vi "labview music visualizer.vi"() -> ()   [LabVIEW 2014]
uses:
  <vilib>/Analysis/3filter.llb/Filter Passband Type.ctl
  <vilib>/sound2/lvsound2.llb/Sampling Mode.ctl
  <vilib>/sound2/lvsound2.llb/Sound Output Write (DBL).vi
  <vilib>/Analysis/3filter.llb/Butterworth Filter (DBL).vi
  <vilib>/sound2/lvsound2.llb/Sound File Read (DBL).vi
  <vilib>/sound2/lvsound2.llb/Sound File Read Open.vi
  <vilib>/sound2/lvsound2.llb/Sound File Info (path).vi
  <vilib>/measure/maspectr.llb/FFT Power Spectrum and PSD for 1 Chan.vi
  <vilib>/measure/NI_MAPro.lvlib
  <vilib>/Analysis/NI_AALBase.lvlib
panel:
  out "Low Cutoff Freq, Hz":u32
  out "High Cutoff Freq, Hz":u32
  out "Filter Error!":bool
  in  "Filter Bands ,Hz":cluster{dbl, dbl}(slide)={22000.0, 10.0} scale=10.0..22000.0
  in  "Filter Type":T1=enum."Bandpass"
  out "Power Spectrum":waveform(dbl)(graph)
  out "digital spectrum":dbl[](array[slide]) scale=-42.0..6.0
  out "VU":dbl(knob) scale=-42.0..6.0
  out "Waveform":waveform(dbl)[](graph)
  in  "Stop":bool
  in  "Buffer Size (samples)":i32=2048
  in  "Music File":path=path "!!!"
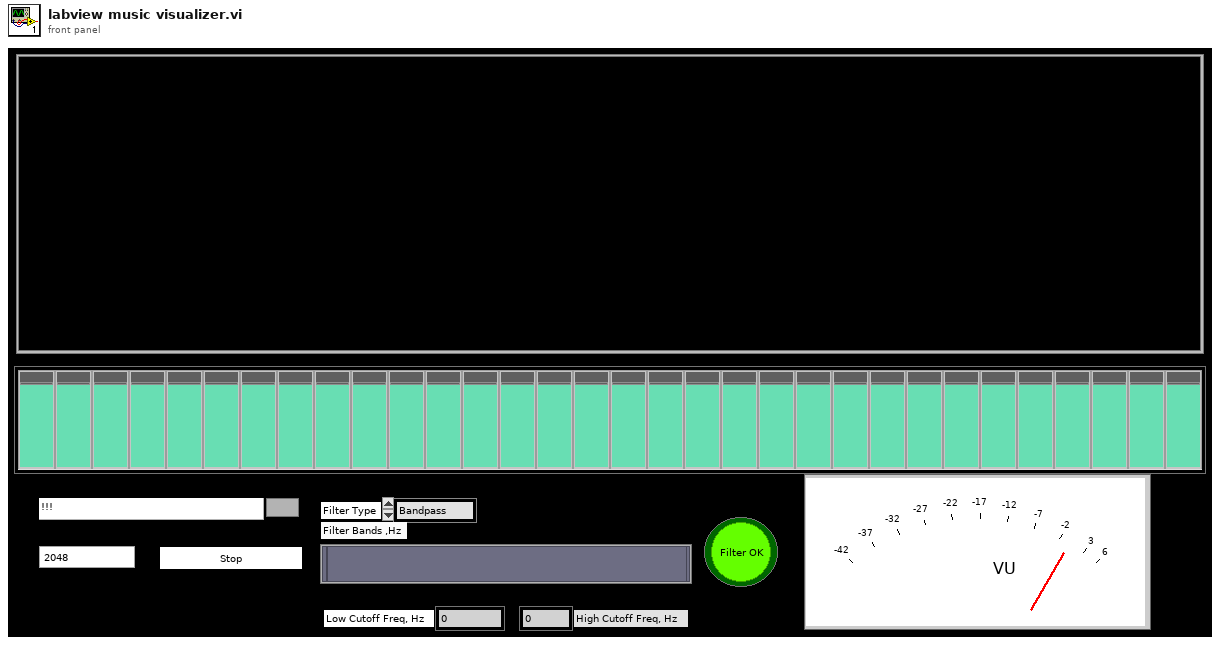
[diagram p1: front panel]
types:
  T1 = typedef "NI_AALBase.lvlib/Filter Passband Type.ctl" = enum32{"Lowpass", "Highpass", "Bandpass", "Bandstop"}
  T2 = typedef "Sampling Mode.ctl" = i32
  T3 = typedef "Sound Data Format.ctl" = cluster{"sample rate (S/s)":dbl, "number of channels":i32, "bits per sample":i32}
  T4 = typedef "Sound Output Task ID.ctl" = u32
  T5 = typedef "Sound File Refnum.ctl" = refnum<file>
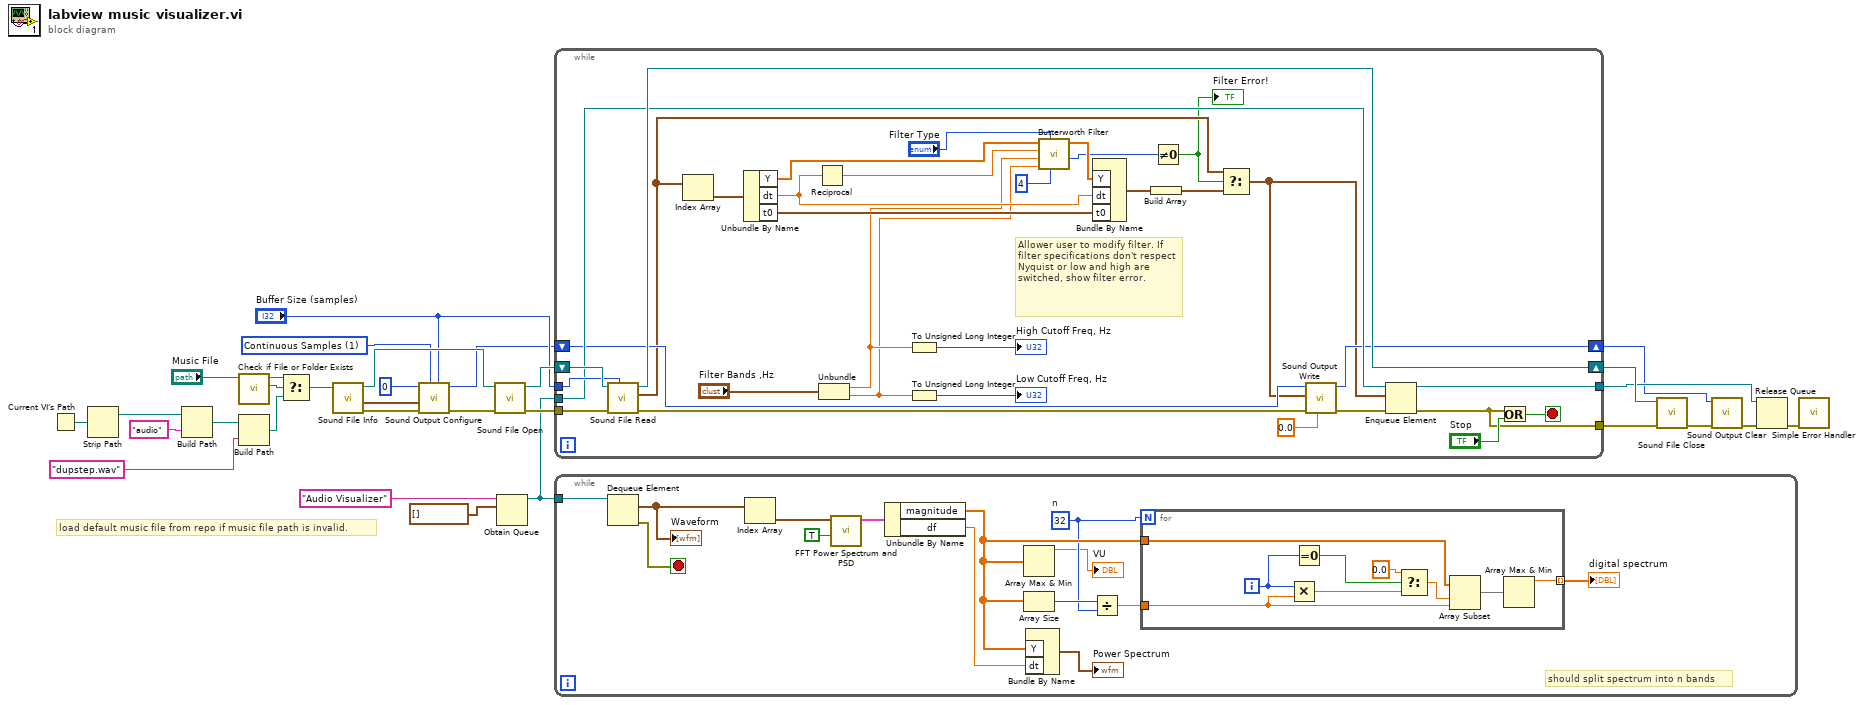
[diagram p0: block diagram]
diagram:
  w11 = T2 1 items=["Finite Samples", "Continuous Samples"] ("sample mode")
  # "load default music file from repo if music file path is invalid."
  n1 = Current VI's Path() -> (path=w10:path)
  n2 = Strip Path(path=w10) -> (stripped path=w9:path)  [unwired: 1 out]
  n3 = Build Path(base path=w9, name or relative path="audio") -> (appended path=w7:path)
  n4 = call <vilib>:"Check if File or Folder Exists.vi"("path"="Music File") -> ("file or folder exists?"=w4:bool, "dup path"=w3:path)  [unwired: 8 in, 1 out]
  n5 = Build Path(base path=w7, name or relative path="dupstep.wav") -> (appended path=w2:path)
  n6 = Select(t=w3, s=w4, f=w2) -> (s? t:f=w1:path)
  n7 = call-poly <vilib>:"Sound File Info.vi"("path"=w1) -> ("error out"=w14:errorcluster, "sound format"=w21:T3, "path out"=w24:path)  [unwired: 7 in, 1 out]
  n8 = call <vilib>:"Sound Output Configure.vi"("number of samples/ch"="Buffer Size (samples)", "sample mode"=w11, "error in (no error)"=w14, "sound format"=w21, "device ID"=u32 0) -> ("error out"=w13:errorcluster, "task ID"=w19:T4)  [unwired: 5 in]
  n9 = call-poly <vilib>:"Sound File Open.vi"("error in (no error)"=w13, "path"=w24) -> ("error out"=w28:errorcluster, "sound file refnum"=w30:T5)  [unwired: 8 in]
  n10 = Obtain Queue(name (unnamed)="Audio Visualizer", element data type=waveform(dbl)[] [] ("data")) -> (queue out=w18:refnum<queue>)  [unwired: 3 in, 2 out]
  n11 = while {
    tunnel: "Buffer Size (samples)" -> [w62]
    shift-right: [w61] -> w29
    shift-left: w30 -> [w63]
    tunnel: w28 -> [w60]
    tunnel: [w56] -> w27
    tunnel: w18 -> [w57]
    tunnel: [w55] -> w26
    shift-right: [w51] -> w15
    shift-left: w19 -> [w54]
    stop <- w59 stop-if-true
    # "Allower user to modify filter. If filter specifications don't respect Nyquist or low and high are switched, show filter error."
    n12 = call-poly <vilib>:"Sound File Read.vi"("number of samples/ch (-1: all)"=w62, "error in (no error)"=w60, "sound file refnum"=w63) -> ("error out"=w53:errorcluster, "data"=w39:waveform(dbl)[], "sound file refnum out"=w61:T5)  [unwired: 4 in, 2 out]
    n13 = Index Array(array=w39) -> (element=w46:waveform(dbl))  [unwired: 1 in]
    n14 = Unbundle By Name(w46) -> ("Y"=w47:dbl[], "dt"=w43:dbl, "t0"=w36:timestamp)
    n15 = Reciprocal(x=w43) -> (1/x=w41:dbl)
    n16 = Unbundle("Filter Bands ,Hz") -> (w34:dbl, w33:dbl)
    n17 = To Unsigned Long Integer(number=w34) -> (unsigned 32bit integer=→"High Cutoff Freq, Hz":u32)
    n18 = To Unsigned Long Integer(number=w33) -> (unsigned 32bit integer=→"Low Cutoff Freq, Hz":u32)
    n19 = call-poly <vilib>:"Butterworth Filter.vi"("order"=4, "filter type"="Filter Type", "low cutoff freq: fl"=w33, "high cutoff freq: fh"=w34, "sampling freq: fs"=w41, "X"=w47) -> ("error"=w40:i32, "Filtered X"=w45:dbl[])  [unwired: 2 in]
    n20 = Bundle By Name("Y"=w45, "dt"=w43, "t0"=w36) -> (w44:waveform(dbl))  [unwired: 1 in]
    n21 = Build Array(w44) -> (w38:waveform(dbl)[])
    n22 = Not Equal To 0?(x=w40) -> (x != 0?=w35:bool)
    "Filter Error!" <- w35
    n23 = Select(t=w39, s=w35, f=w38) -> (s? t:f=w37:waveform(dbl)[])
    n24 = call-poly <vilib>:"Sound Output Write.vi"("timeout (sec)"=0.0, "error in (no error)"=w53, "data"=w37, "task ID"=w54) -> ("error out"=w52:errorcluster, "task ID out"=w51:T4)  [unwired: 6 in]
    n25 = Enqueue Element(queue=w57, element=w37, error in (no error)=w52) -> (queue out=w55:refnum<queue>, error out=w56:errorcluster)  [unwired: 1 in, 1 out]
    n26 = Or(x=w56, y="Stop") -> (x .or. y?=w59:bool)
  }
  n27 = while {
    tunnel: w18 -> [w77]
    stop <- w76 stop-if-true
    w66 = 32  # n
    # "should split spectrum into n bands"
    n28 = Dequeue Element(queue=w77) -> (element=w75:waveform(dbl)[], error out=w76:errorcluster)  [unwired: 2 in, 2 out]
    "Waveform" <- w75
    n29 = Index Array(array=w75) -> (element=w74:waveform(dbl))  [unwired: 1 in]
    n30 = call-poly <vilib>:"FFT Power Spectrum and PSD.vi"("dB On (F)"=TRUE, "time signal"=w74) -> ("Power Spectrum / PSD"=w72:cluster{"f0":dbl, "df":dbl, "magnitude":dbl[]})  [unwired: 6 in, 3 out]
    n31 = Unbundle By Name(w72) -> ("magnitude"=w67:dbl[], "df"=w71:dbl)
    n32 = Array Max & Min(array=w67) -> (max value=→"VU":dbl)  [unwired: 3 out]
    n33 = Array Size(array=w67) -> (size(s)=w69:i32)
    n34 = Bundle By Name("Y"=w67, "dt"=w71) -> (→"Power Spectrum":waveform(dbl))  [unwired: 1 in]
    n35 = Divide(x=w69, y=w66) -> (x/y=w68:dbl)
    n36 = for {
      N: w66 -> [_]
      tunnel: w68 -> [w80]
      tunnel: w67 -> [w86]
      tunnel: [w78] -> w64 mode=indexing
      i -> [w83]
      n37 = Multiply(x=w83, y=w80) -> (x*y=w82:dbl)
      n38 = Equal To 0?(x=w83) -> (x = 0?=w85:bool)
      n39 = Select(t=0.0, s=w85, f=w82) -> (s? t:f=w81:dbl)
      n40 = Array Subset(array=w86, index=w81, length=w80) -> (w79:dbl[])
      n41 = Array Max & Min(array=w79) -> (max value=w78:dbl)  [unwired: 3 out]
    }
    "digital spectrum" <- w64
  }
  n42 = call <vilib>:"Sound File Close.vi"("error in (no error)"=w27, "sound file refnum"=w29) -> ("error out"=w17:errorcluster)  [unwired: 9 in]
  n43 = call <vilib>:"Sound Output Clear.vi"("error in (no error)"=w17, "task ID"=w15) -> ("error out"=w16:errorcluster)  [unwired: 9 in]
  n44 = Release Queue(queue=w26, error in (no error)=w16) -> (error out=w25:errorcluster)  [unwired: 1 in, 2 out]
  n45 = call <vilib>:"Simple Error Handler.vi"("error in (no error)"=w25) -> ()  [unwired: 4 in, 5 out]
